vi "Format Into String Multiple.vi"(8 "error in":errorcluster, 10 "Format String":string, 11 "Input Values":variant) -> (0 "error out":errorcluster, 3 "Formated String":string)   [LabVIEW 2021]
doc: "Takes multiple inputs from <b>Input Values</b> (cluster, array or element) and tries to format them into the <b>Format String</b> input. The input cluster can also contain multiple clusters and arrays. The <b>Input Values</b> data types and order must match the types and order of the formatting symbols in <b>Format String</b> input. \nIf the <b>Include Call Chain?</b> is True then the call chain of the error is appended to the end of <b>Formatted Output</b>.\n\nFormated output is returned at <b>Formated Output</b>"
uses:
  <vilib>/Utility/Data Type/NI_Data Type.lvlib
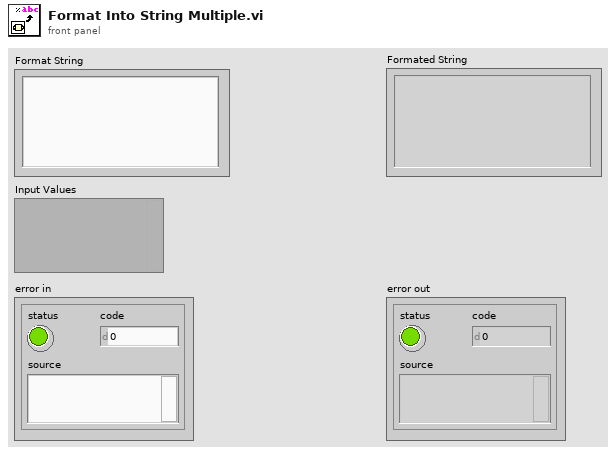
[diagram p1: front panel]
types:
  T1 = typedef "NI_Data Type.lvlib/Data Type.ctl" = enum8{"Invalid Type", "Void", "I8", "I16", "I32", "I64", "U8", "U16", "U32", "U64", "Single Float", "Double Float", "Extended Float", "Single Complex", "Double Complex", "Extended Complex", "Enum U8", "Enum U16", "Enum U32", "Enum U64", "Single Float With Unit", "Double Float With Unit", "Extended Float With Unit", "Single Complex with Unit", "Double Complex with Unit", "Extended Complex with Unit", "Boolean", "String", "Path", "Picture", "Tag", "Array", "Cluster", "Variant", "LV Variant", "Waveform", "Timestamp", "Digital Waveform", "Digital Data", "ExpressData", "Refnum", "External Data", "VI", "Poly VI", "LabVIEW Class Instance", "Fixed Point", "Set Collection", "Map Collection"}
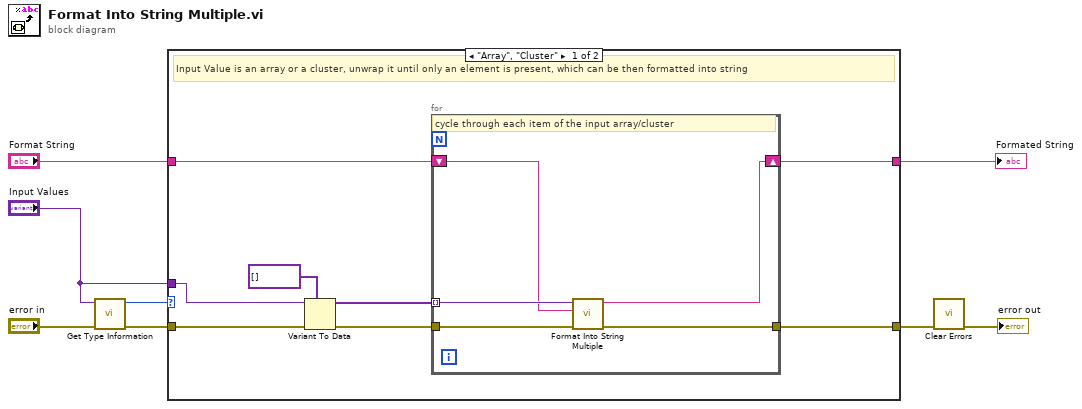
[diagram p0: block diagram]
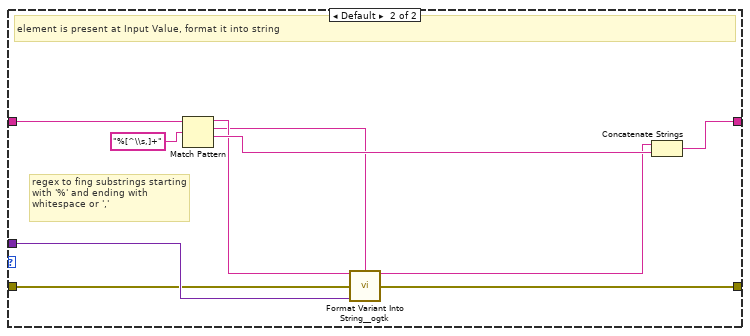
[diagram p2: hidden frame]
diagram:
  n1 = call <vilib>:"Get Type Information.vi"("error in (no error)"="error in", "variant"="Input Values") -> ("error out"=w7:errorcluster, "type"=w6:T1)  [unwired: 5 in, 3 out]
  n2 = case shown="\"Array\", \"Cluster\"" w6 {
    tunnel: w7 -> [w15 w23]
    tunnel: "Input Values" -> [w14 w24]
    tunnel: "Format String" -> [w11 w26]
    tunnel: [w10 w25] -> w3
    tunnel: [w9 w22] -> w2
    frame "Array", "Cluster" {
      # "Input Value is an array or a cluster, unwrap it until only an element is present, which can be then formatted into string"
      n3 = Variant To Data(error in=w15, type=variant[] [], Variant=w14) -> (data=w13:variant[], error out=w12:errorcluster)
      n4 = for {
        tunnel: w13 -> [w21] mode=indexing
        shift-right: [w18] -> w10
        shift-left: w11 -> [w19]
        tunnel: w12 -> [w20]
        tunnel: [w17] -> w9
        # "cycle through each item of the input array/cluster"
        n5 = call "Format Into String Multiple.vi"("error in"=w20, "Format String"=w19, "Input Values"=w21) -> ("error out"=w17:errorcluster, "Formated String"=w18:string)  [unwired: 7 in]
      }
    }
    frame Default {
      # "regex to fing substrings starting with '%' and ending with whitespace or ','"
      # "element is present at Input Value, format it into string"
      n6 = Match Pattern(string=w26, regular expression="%[^\\s,]+") -> (before substring=w29:string, match substring=w28:string, after substring=w30:string)  [unwired: 1 in, 1 out]
      n7 = call <userlib>:"Format Variant Into String__ogtk.vi"("Input String"=w29, "Format String"=w28, "error in (no error)"=w23, "Variant"=w24) -> ("Output String"=w27:string, "error out"=w22:errorcluster)  [unwired: 10 in]
      n8 = Concatenate Strings(w27, w30) -> (w25:string)
    }
  }
  "Formated String" <- w3
  n9 = call <vilib>:"Clear Errors.vi"("error in (no error)"=w2) -> ("error out"=→"error out":errorcluster)  [unwired: 5 in, 1 out]
